vi "Protocol.Output Messages.vi"(8 "error in (no error)":errorcluster, 11 "J1939 Main Configuration":T1 {"Stream Refs"."Termination" items=["Off", "On"]}) -> (0 "error out":errorcluster)   [LabVIEW 2019, in "J1939 Addon Engine.lvlib"]
uses:
  J1939 Addon Engine.lvlib
  Types/Protocol.Configuration.ctl
  <vilib>/NI/NI VeriStand Addon Network Comm/Engine/VeriStand Comm.lvclass
  <vilib>/NI/NIVS Inline Async API/_VS Inline Async API/Process/Process.lvclass
  Types/Protocol.Refs.ctl
  Support Libraries/J1939 Utilities/Types/CAN Outgoing Message Cluster.ctl
  Types/Protocol.RQST Lookup Table Reference.ctl
  Types/Protocol.Address Table Reference.ctl
  Types/Protocol.XNET Settings.ctl
  <vilib>/NI/NIVS Inline Async API/_Data Access Engine/Data Access Engine/Types/Read.DVR.ctl
  <vilib>/NI/NIVS Inline Async API/_Data Access Engine/Access Type Classes/Read/Read.lvclass
  <vilib>/NI/NIVS Inline Async API/_Data Access Engine/Data Access Engine/Types/Write.DVR.ctl
  <vilib>/NI/NIVS Inline Async API/_Data Access Engine/Access Type Classes/Write/Write.lvclass
  Types/CounterAndProtectionFrames.ctl
  SubModules/Frame-Protection-Support/Source/Engine/Types/RT Frame Settings.ctl
  SubModules/Frame-Protection-Support/Source/Shared/Types/Exported Frame Type.ctl
  SubModules/Frame-Protection-Support/Source/Engine/Types/RT Protection Configuration.ctl
  SubModules/Frame-Protection-Support/Source/Shared/Types/Protection Type.ctl
  SubModules/Frame-Protection-Support/Source/Shared/Types/XNET Signal Configuration.ctl
  SubModules/Frame-Protection-Support/Source/Shared/Types/Exported Counter Settings.ctl
  SubModules/Frame-Protection-Support/Source/Shared/Types/Exported Event Trigger Type.ctl
  SubModules/CAN-Streaming-Support/Addon/Addon Engine/Types/Engine Stream Refs.ctl
  SubModules/CAN-Streaming-Support/Addon/Addon Shared/Types/Direction Filter.ctl
  SubModules/CAN-Streaming-Support/Addon/Addon Shared/Types/Type Filter.ctl
  SubModules/CAN-Streaming-Support/Addon/Addon Shared/Types/Filter Parameters.ctl
  <vilib>/Platform/TimedLoop/XDataNode/timing_clust.ctl
  <vilib>/Platform/TimedLoop/XDataNode/nitl_modes.ctl
  <vilib>/Platform/TimedLoop/XDataNode/wakeup.ctl
  <vilib>/NI/NIVS Inline Async API/_Data Access Engine/Access Type Classes/Read/Read.lvclass/Read.ctl
  <vilib>/NI/NIVS Inline Async API/_Data Access Engine/Access Type Classes/Write/Write.lvclass/Write.ctl
  <vilib>/NI/NIVS Inline Async API/_VS Inline Async API/Process/Process.lvclass/Process.ctl
  <vilib>/NI/NIVS Inline Async API/_VS Inline Async API/Error Handling Process/SubVIs/Error.ConvertArray.vi
  <vilib>/NI/NIVS Inline Async API/_Data Access Engine/Data Access Engine/Methods/Data.Processes.Execute.vi
  <vilib>/NI/NIVS Inline Async API/_Data Access Engine/Data Access Engine/Methods/Read.Data.Detect.vi
  SubModules/Frame-Protection-Support/Source/Engine/SubVIs/Determine Transmit.vi
  SubModules/Frame-Protection-Support/Source/Engine/SubVIs/Update Counter Signals.vi
  SubModules/Frame-Protection-Support/Source/Engine/SubVIs/Get Frame Data.vi
  SubModules/Frame-Protection-Support/Source/Engine/SubVIs/Convert EU Data to XNET Frame.vi
  SubModules/Frame-Protection-Support/Source/Engine/SubVIs/Update Protection Signals.vi
  SubModules/Frame-Protection-Support/Source/Engine/SubVIs/Determine Disabled.vi
  <vilib>/NI/NIVS Inline Async API/_Data Access Engine/Data Access Engine/Methods/Write.Data.Commit.vi
  <vilib>/NI/NIVS Inline Async API/_Data Access Engine/Access Type Classes/Read/Read.ProcessData.Detect.vi
  SubModules/Frame-Protection-Support/Source/Engine/SubVIs/Determine Transmission.vi
  SubModules/Frame-Protection-Support/Source/Engine/SubVIs/Determine Periodic.vi
  SubModules/Frame-Protection-Support/Source/Engine/SubVIs/Set Counter Signal.vi
  SubModules/Frame-Protection-Support/Source/Engine/SubVIs/Calculate Counter Value.vi
  SubModules/Frame-Protection-Support/Source/Engine/SubVIs/Set Protection Signal.vi
  SubModules/Frame-Protection-Support/Source/Engine/SubVIs/Calculate Protection Value.vi
  <vilib>/NI/NIVS Inline Async API/_Data Access Engine/Access Type Classes/Write/Write.Commit.vi
  <vilib>/NI/NIVS Inline Async API/_Data Access Engine/Data Access Engine/Methods/Write.Data.Buffer.vi
  SubModules/Frame-Protection-Support/Source/Engine/SubVIs/Get Protection Signals.vi
  <vilib>/NI/NIVS Inline Async API/_Data Access Engine/Access Type Classes/Write/Write.Buffer.vi
  <vilib>/xnet/xnet.llb/XNET Convert.vi
  <vilib>/xnet/xnet.llb/XNET Convert (Signal to Frame Raw).vi
  <vilib>/xnet/xnet.llb/XNET Convert (Signal to Frame CAN).vi
  <vilib>/xnet/xnet.llb/XNET Write (Frame CAN).vi
  <vilib>/Platform/TimedLoop/XDataNode/XDataNode.xnode
  SubModules/Frame-Protection-Support/Source/Engine/Protection and Counter Support Engine.lvlib
  <vilib>/Platform/TimedLoop/XDataNode/XDNodeRunTimeDep.lvlib
  Support Libraries/J1939 Utilities/J1939 Utilities.lvlib
  <vilib>/NI/NIVS Inline Async API/_Data Access Engine/Data Access Engine/Data Access Engine.lvclass
  SubModules/Frame-Protection-Support/Source/Shared/Protection and Counter Support Shared.lvlib
  SubModules/CAN-Streaming-Support/Addon/Addon Shared/CAN Stream Support Shared.lvlib
  SubModules/CAN-Streaming-Support/Addon/Addon Engine/CAN Stream Support Engine.lvlib
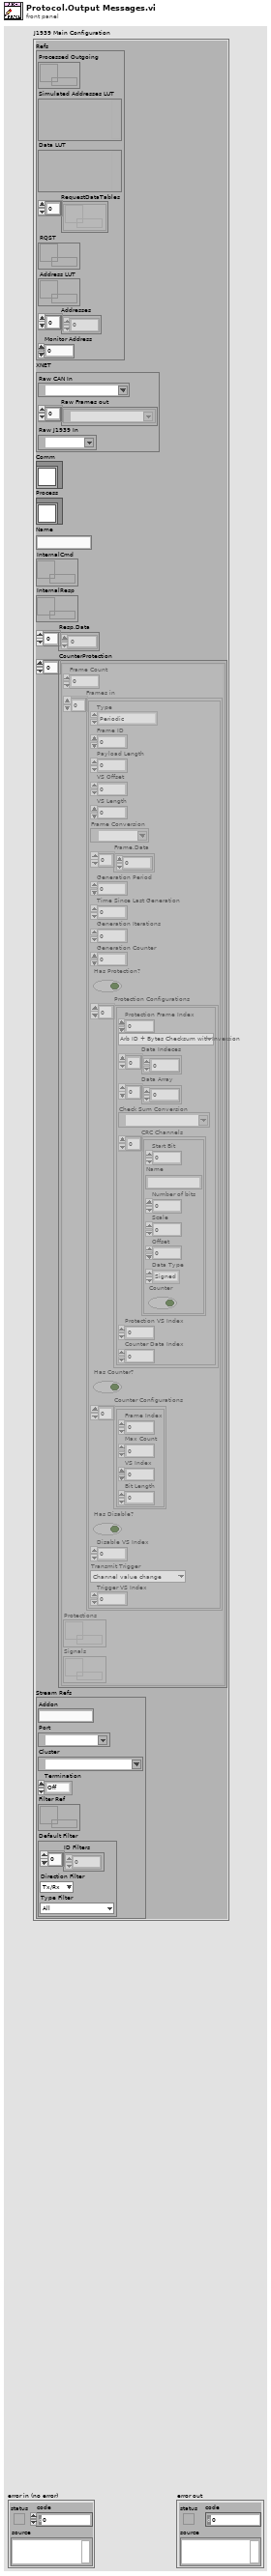
[diagram p1: front panel]
types:
  T1 = typedef "J1939 Addon Engine.lvlib/Protocol.Configuration.ctl" = cluster{"Refs":T2, "XNET":T5, "Comm":refnum<class "VeriStand Comm.lvclass">, "Process":refnum<class "Process.lvclass">, "Name":string, "InternalCmd":T6, "InternalResp":T7, "Resp.Data":dbl[], "CounterProtection":T8[], "Stream Refs":T16}
  T2 = typedef "J1939 Addon Engine.lvlib/Protocol.Refs.ctl" = cluster{"Processed Outgoing":refnum<queue>, "Simulated Addresses LUT":variant, "Data LUT":variant, "RequestDataTables":refnum<k33>[], "RQST":T3, "Address LUT":T4, "Addresses":u8[], "Monitor Address":u8}
  T3 = typedef "J1939 Addon Engine.lvlib/Protocol.RQST Lookup Table Reference.ctl" = refnum<data-value>
  T4 = typedef "J1939 Addon Engine.lvlib/Protocol.Address Table Reference.ctl" = refnum<data-value>
  T5 = typedef "J1939 Addon Engine.lvlib/Protocol.XNET Settings.ctl" = cluster{"Raw CAN In":refnum<k21>, "Raw Frames out":refnum<k21>[], "Raw J1939 In":refnum<k21>}
  T6 = typedef "Data Access Engine.lvlib/Data Access Engine.lvclass/Read.DVR.ctl" = refnum<data-value>
  T7 = typedef "Data Access Engine.lvlib/Data Access Engine.lvclass/Write.DVR.ctl" = refnum<data-value>
  T8 = typedef "J1939 Addon Engine.lvlib/CounterAndProtectionFrames.ctl" = cluster{"Frame Count":i32, "Frames in":T9[], "Protections":T7, "Signals":T6}
  T9 = typedef "Protection and Counter Support Engine.lvlib/RT Frame Settings.ctl" = cluster{"Type":T10, "Frame ID":u32, "Payload Length":u32, "VS Offset":i32, "VS Length":i32, "Frame Conversion":refnum<k21>, "Frame.Data":dbl[], "Generation Period":u32, "Time Since Last Generation":u32, "Generation Iterations":u32, "Generation Counter":u32, "Has Protection?":bool, "Protection Configurations":T11[], "Has Counter?":bool, "Counter Configurations":T14[], "Has Disable?":bool, "Disable VS Index":i32, "Transmit Trigger":T15, "Trigger VS Index":i32}
  T10 = typedef "Protection and Counter Support Shared.lvlib/Exported Frame Type.ctl" = enum16{"Periodic", "Event", "Periodic/Event"}
  T11 = typedef "Protection and Counter Support Engine.lvlib/RT Protection Configuration.ctl" = cluster{"Protection Frame Index":i32, "Protection Type":T12, "Data Indeces":i32[], "Data Array":dbl[], "Check Sum Conversion":refnum<k21>, "CRC Channels":T13[], "Protection VS Index":i32, "Counter Data Index":i32}
  T12 = typedef "Protection and Counter Support Shared.lvlib/Protection Type.ctl" = enum16{"Arb ID + Bytes Checksum with Inversion", "Arb ID + Bytes CRC with Inversion", "Reversed Raw Signal Checksum with Inversion", "Concatenated Two's Compliment"}
  T13 = typedef "Protection and Counter Support Shared.lvlib/XNET Signal Configuration.ctl" = cluster{"Start Bit":i32, "Name":string, "Number of bits":i32, "Scale":dbl, "Offset":dbl, "Data Type":u32, "Counter":bool}
  T14 = typedef "Protection and Counter Support Shared.lvlib/Exported Counter Settings.ctl" = cluster{"Frame Index":i32, "Max Count":dbl, "VS Index":i32, "Bit Length":i64}
  T15 = typedef "Protection and Counter Support Shared.lvlib/Exported Event Trigger Type.ctl" = enum16{"Channel value change", "Trigger channel (not zero)", "Channel value change or trigger channel (not zero)", "Trigger channel (any value change)", "Channel value change or trigger channel (any value change)"}
  T16 = typedef "CAN Stream Support Engine.lvlib/Engine Stream Refs.ctl" = cluster{"Addon":string, "Port":refnum<k21>, "Cluster":refnum<k21>, "Termination":u32, "Filter Ref":refnum<data-value>, "Default Filter":T17}
  T17 = typedef "CAN Stream Support Shared.lvlib/Filter Parameters.ctl" = cluster{"ID Filters":u32[], "Direction Filter":T18, "Type Filter":T19}
  T18 = typedef "CAN Stream Support Shared.lvlib/Direction Filter.ctl" = enum16{"Tx/Rx", "Rx", "Tx"}
  T19 = typedef "CAN Stream Support Shared.lvlib/Type Filter.ctl" = enum16{"All", "CAN Data", "CAN Remote", "CAN Bus Error", "CAN 2.0 Data", "CAN FD Data", "CAN FD+BRS Data", "J1939 Data", "Delay", "Log Trigger", "Start Trigger"}
  T20 = typedef "XDNodeRunTimeDep.lvlib/timing_clust.ctl" = cluster{"Expected End [f-1]":u64, "Actual End [f-1]":u64, "Finished Late? [f-1]":bool, "Expected End [i-1]":u64, "Actual End [i-1]":u64, "Finished Late? [i-1]":bool, "Expected Start [i]":u64, "Actual Start [i]":u64, "Expected Start [f]":u64, "Actual Start [f]":u64, "Source Name":string, "Structure Name":string, "Period":i64, "Deadline":i64, "Offset":i64, "Start":i64, "Priority":i32, "Timeout":i32, "Mode":T21, "Wakeup Reason":T22, "Error":errorcluster, "Source Type":string, "Secondary Source Type":string, "Global End Time":u64, "Global Start Time":u64, "Frame Duration":u64, "Iteration Duration":u64, "Assigned CPU":i32, "I/O Scan Engine Mode":u32}
  T21 = typedef "XDNodeRunTimeDep.lvlib/nitl_modes.ctl" = enum32{"No Change", "Process missed periods, maintain original phase", "Discard missed periods, maintain original phase", "Process missed periods, ignore original phase", "Discard missed periods, ignore original phase"}
  T22 = typedef "XDNodeRunTimeDep.lvlib/wakeup.ctl" = enum32{"Normal", "Aborted", "Asynchronous wakeup", "Timing source error", "Timed loop error", "Timeout"}
  T23 = typedef "XNET Frame CAN.ctl" = cluster{"timestamp":timestamp, "payload":u8[], "identifier":u32, "type":T24, "extended?":bool, "echo?":bool}
  T24 = typedef "XNET Frame Type CAN.ctl" = u8
  T25 = typedef "J1939 Utilities.lvlib/CAN Outgoing Message Cluster.ctl" = cluster{"Identifier":u32, "Data":u8[]}
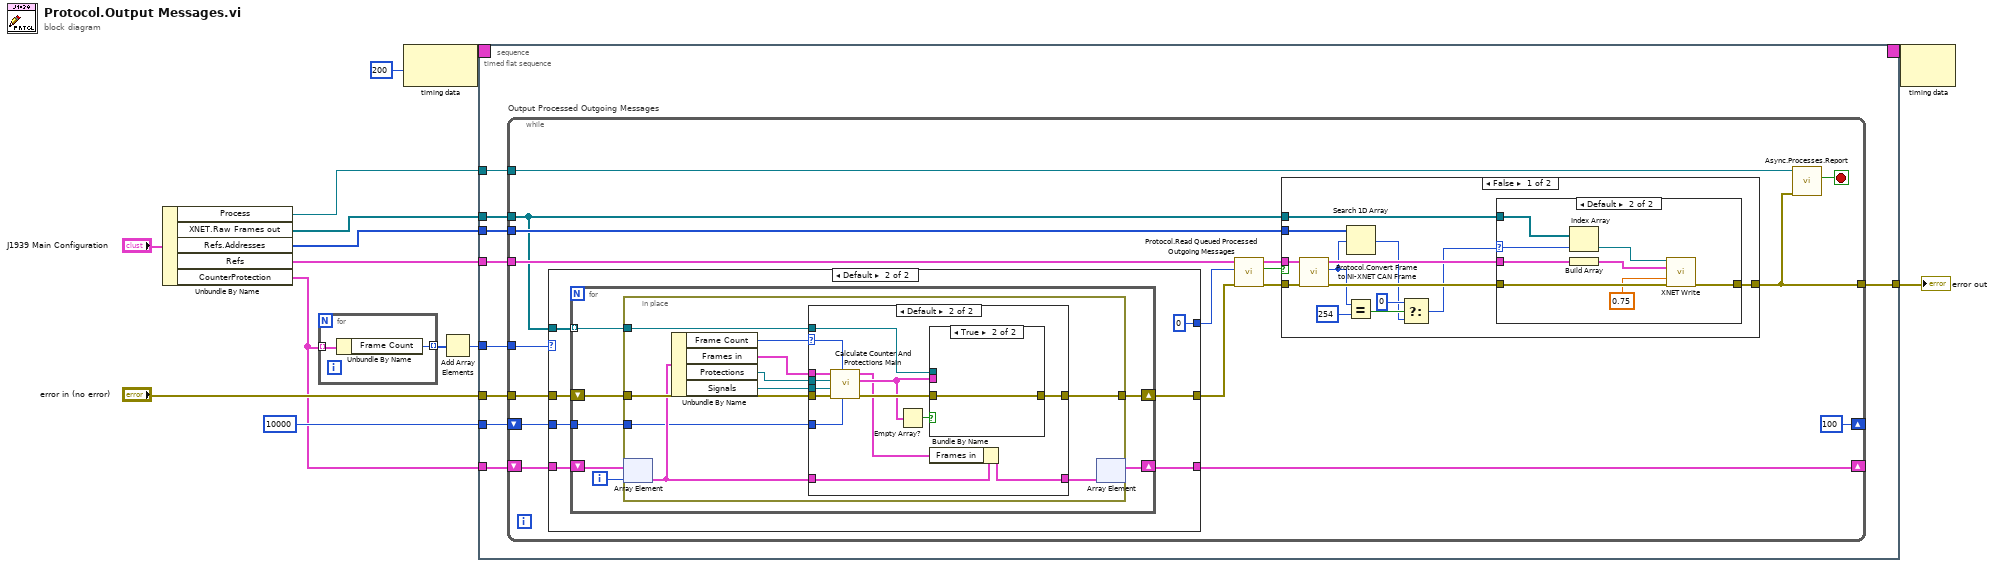
[diagram p0: block diagram]
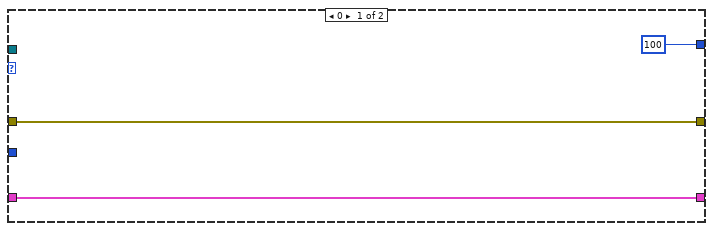
[diagram p2: hidden frame]
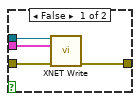
[diagram p4: hidden frame]
diagram:
  n1 = Unbundle By Name("J1939 Main Configuration") -> ("Process"=w14:refnum<class "Process.lvclass">, "XNET.Raw Frames out"=w13:refnum<k21>[], "Refs.Addresses"=w8:u8[], "Refs"=w12:T2, "CounterProtection"=w3:T8[])
  n2 = for {
    tunnel: w3 -> [w16] mode=indexing
    tunnel: [w15] -> w2 mode=indexing
    n3 = Unbundle By Name(w16) -> ("Frame Count"=w15:i32)
  }
  n4 = node-c288(200 ("Priority")) -> (w7:T20)
  n5 = Add Array Elements(numeric array=w2) -> (sum=w1:i32)
  n6 = timed-sequence {
    timing: w7 -> [_]
    timing-out: [_] -> w6
    tunnel: w14 -> [w25]
    tunnel: w13 -> [w24]
    tunnel: w12 -> [w23]
    tunnel: "error in (no error)" -> [w22]
    tunnel: [w21] -> w9
    tunnel: w8 -> [w20]
    tunnel: w3 -> [w19]
    tunnel: 10000 -> [w18]
    tunnel: w1 -> [w17]
    n7 = timed-flat-sequence {
      tunnel: w25 -> [w34]
      tunnel: w24 -> [w33]
      tunnel: w23 -> [w32]
      tunnel: w22 -> [w31]
      tunnel: [w30] -> w21
      tunnel: w20 -> [w29]
      tunnel: w19 -> [w28]
      tunnel: w18 -> [w27]
      tunnel: w17 -> [w26]
      n8 = while "Output Processed Outgoing Messages" {
        tunnel: w32 -> [w51]
        tunnel: w31 -> [w41]
        tunnel: [w42] -> w30
        tunnel: w33 -> [w39]
        tunnel: w34 -> [w45]
        tunnel: w29 -> [w47]
        shift-right: [w43] -> _
        shift-left: w28 -> [w44]
        shift-right: [100] -> _
        shift-left: w27 -> [w38]
        tunnel: w26 -> [w36]
        stop <- w46 stop-if-true
        n9 = case shown="Default" w36 {
          tunnel: w44 -> [w54 w61]
          tunnel: [w54 w60] -> w43
          tunnel: w41 -> [w53 w59]
          tunnel: [w53 w58] -> w40
          tunnel: w39 -> [_ w57]
          tunnel: w38 -> [_ w56]
          tunnel: [100 ("timeout in ms (-1)") 0 ("timeout in ms (-1)")] -> w35
          frame 0 {
          }
          frame Default {
            n10 = for {
              shift-right: [w67] -> w58
              shift-left: w59 -> [w68]
              tunnel: w57 -> [w66] mode=indexing
              shift-right: [w63] -> w60
              shift-left: w61 -> [w64]
              tunnel: w56 -> [w62]
              i -> [w65]
              n11 = in-place {
                in-place-border: w68 -> [w78]
                in-place-border: [w77] -> w67
                in-place-border: w66 -> [w76]
                in-place-border: w62 -> [w69]
                n12 = in-place-array #1(w64, w65) -> (w72:T8)
                n13 = Unbundle By Name(w72) -> ("Frame Count"=w70:i32, "Frames in"=w75:T9[], "Protections"=w74:T7, "Signals"=w73:T6)
                n14 = case shown="Default" w70 {
                  selector: w70 -> [_ w82]
                  tunnel: w78 -> [w80 w94]
                  tunnel: [w80 w93] -> w77
                  tunnel: w76 -> [_ w92]
                  tunnel: w75 -> [_ w88]
                  tunnel: w74 -> [_ w87]
                  tunnel: w73 -> [_ w86]
                  tunnel: w72 -> [w79 w85]
                  tunnel: [w79 w83] -> w71
                  tunnel: w69 -> [_ w81]
                  frame 0 {
                  }
                  frame Default {
                    n15 = call "Calculate Counter And Protections Main.vi"("timeout ms"=w81, "Frame Count"=w82, "error in (no error)"=w94, "Signals"=w86, "Protections"=w87, "Frames in"=w88) -> ("error out"=w91:errorcluster, "Frames"=w90:T23[], "Frames out"=w84:T9[])  [unwired: 2 in, 1 out]
                    n16 = Empty Array?(array=w90) -> (empty?=w89:bool)
                    n17 = case shown="True" w89 {
                      tunnel: [w98 w99] -> w93
                      tunnel: w92 -> [w97 _]
                      tunnel: w91 -> [w96 w99]
                      tunnel: w90 -> [w95 _]
                      frame False {
                        n18 = call-poly <vilib>:"XNET Write.vi"("session in"=w97, "data"=w95, "error in (no error)"=w96) -> ("error out"=w98:errorcluster)  [unwired: 12 out]
                      }
                      frame True {
                      }
                    }
                    n19 = Bundle By Name(cluster=w85, "Frames in"=w84) -> (w83:T8)
                  }
                }
                n20 = in-place-array #1(w71) -> (w63:T8[])  [unwired: 1 out]
              }
            }
          }
        }
        n21 = call "Protocol.Read Queued Processed Outgoing Messages.vi"("error in (no error)"=w40, "timeout in ms (-1)"=w35, "J1939 Cluster"=w51) -> ("error out"=w50:errorcluster, "timed out?"=w48:bool, "Frame"=w49:T25)  [unwired: 6 in]
        n22 = case shown="False" w48 {
          tunnel: w50 -> [w100 w122]
          tunnel: w49 -> [w112 _]
          tunnel: w39 -> [w107 _]
          tunnel: [w111 w122] -> w42
          tunnel: w47 -> [w108 _]
          frame False {
            n23 = call "Protocol.Convert Frame to NI-XNET CAN Frame.vi"("error in (no error)"=w100, "Data to Send"=w112) -> ("error out"=w109:errorcluster, "Source Address"=w102:u8, "CAN frame"=w110:T23)  [unwired: 7 out]
            n24 = Search 1D Array(1D array=w108, element=w102) -> (index of element=w101:i32)  [unwired: 1 in]
            n25 = Equal?(x=w102, y=u8 254) -> (x = y?=w105:bool)
            n26 = Select(t=0, s=w105, f=w101) -> (s? t:f=w103:i32)
            n27 = case shown="Default" w103 {
              selector: w103 -> [_ w116]
              tunnel: [w113 w121] -> w111
              tunnel: w110 -> [_ w120]
              tunnel: w109 -> [w113 w119]
              tunnel: w107 -> [_ w114]
              frame -1 {
              }
              frame Default {
                n28 = Index Array(array=w114, index=w116) -> (element=w117:refnum<k21>)
                n29 = Build Array(w120) -> (w115:T23[])
                n30 = call-poly <vilib>:"XNET Write.vi"("session in"=w117, "data"=w115, "timeout (10)"=0.75, "error in (no error)"=w119) -> ("error out"=w121:errorcluster)  [unwired: 11 out]
              }
            }
          }
          frame True {
          }
        }
        n31 = call <vilib>:"Async.Processes.Report.vi"("Error"=w42, "Process in"=w45) -> ("Stop"=w46:bool)  [unwired: 8 in, 1 out]
      }
    }
  }
  "error out" <- w9
  n32 = node-c288(w6) -> ()  [unwired: 1 out]
